vi "Tosca-Create And Enqueue Stimulus Rep.vi"(0 "Stim data in":T1, 1 "AODO Queue":refnum<queue>, 5 "Nreps":i32, 7 "Nqueue in":i32, 9 "Rep":i32, 11 "error in (no error)":errorcluster, 13 "tail":dbl[][](array[numeric])) -> (4 "Stim data out":T1, 8 "Nqueue out":i32, 15 "error out":errorcluster)   [LabVIEW 2020]
uses:
  Typedefs/Tosca-State AODO.ctl
  epl-vi-lib/Signal Synthesis VIs/4th Generation/Classes/SignalManager/SignalManager.lvclass
  Typedefs/Tosca-AO Runtime.ctl
  Typedefs/Tosca-DO Runtime.ctl
  Typedefs/Tosca-AODO Data.ctl
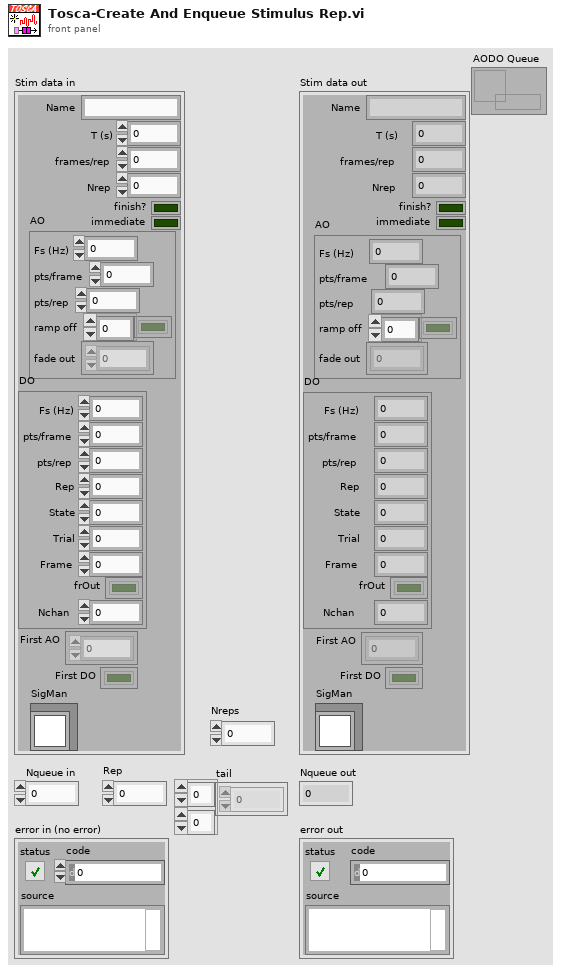
[diagram p1: front panel]
types:
  T1 = typedef "Tosca-State AODO.ctl" = cluster{"Name":string, "T (s)":dbl, "First AO":dbl[][], "frames/rep":i32, "finish?":bool, "Nrep":i32, "AO":T2, "DO":T3, "immediate":bool, "First DO":bool[][], "SigMan":refnum<class "SignalManager.lvclass">}
  T2 = typedef "Tosca-AO Runtime.ctl" = cluster{"Fs (Hz)":dbl, "pts/frame":i32, "pts/rep":i32, "ramp off":bool[], "fade out":dbl[][]}
  T3 = typedef "Tosca-DO Runtime.ctl" = cluster{"Fs (Hz)":dbl, "pts/frame":i32, "pts/rep":i32, "Rep":i32, "State":i32, "Trial":i32, "Frame":i32, "frOut":bool[], "Nchan":i32}
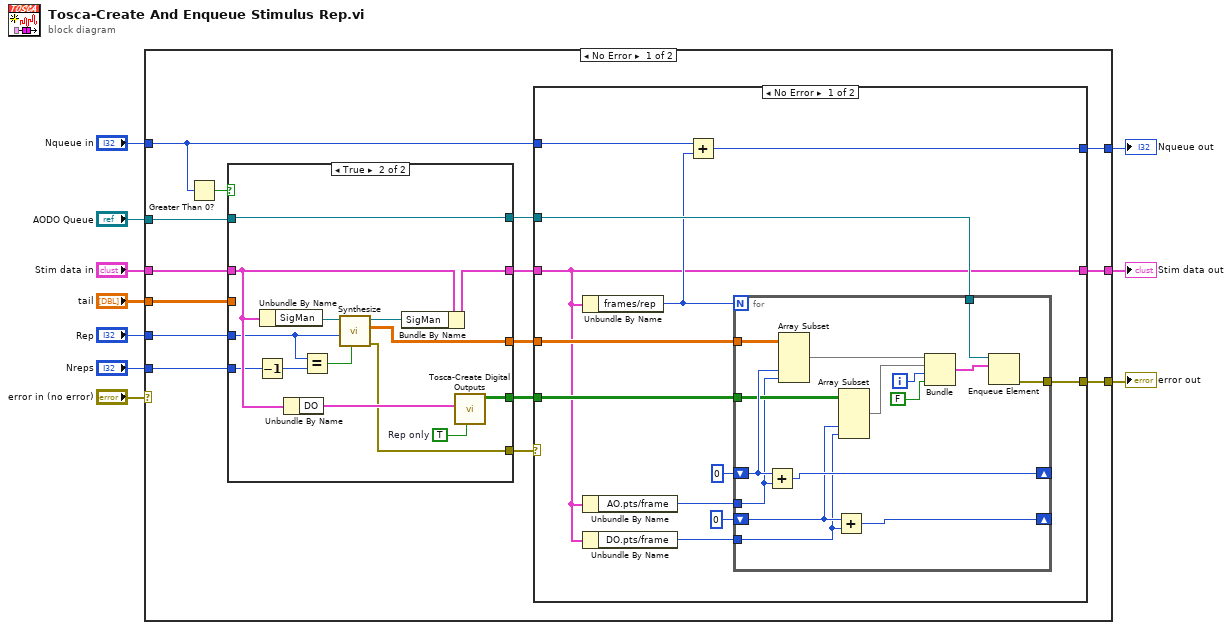
[diagram p0: block diagram]
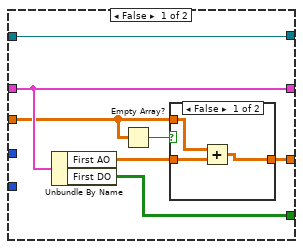
[diagram p3: hidden frame]
diagram:
  n1 = case shown="No Error" "error in (no error)" {
    selector: "error in (no error)" -> [_ w83]
    tunnel: "Stim data in" -> [w25 w81]
    tunnel: "Rep" -> [w24 _]
    tunnel: [w16 w81] -> w8
    tunnel: "AODO Queue" -> [w13 _]
    tunnel: "Nqueue in" -> [w20 w82]
    tunnel: [w19 w82] -> w5
    tunnel: [w18 w83] -> w4
    tunnel: "tail" -> [w12 _]
    tunnel: "Nreps" -> [w11 _]
    frame No Error {
      n2 = Greater Than 0?(x=w20) -> (x > 0?=w15:bool)
      n3 = case shown="True" w15 {
        tunnel: w25 -> [w60 w73]
        tunnel: [w56 w71] -> w23
        tunnel: [w62 w75] -> w21
        tunnel: [w60 w78] -> w22
        tunnel: [_ w74] -> w17
        tunnel: w24 -> [_ w70]
        tunnel: [w61 w72] -> w14
        tunnel: w13 -> [w61 w72]
        tunnel: w12 -> [w58 _]
        tunnel: w11 -> [_ w69]
        frame False {
          n4 = Unbundle By Name(w60) -> ("First AO"=w57:dbl[][], "First DO"=w62:bool[][])
          n5 = Empty Array?(array=w58) -> (empty?=w59:bool)
          n6 = case shown="False" w59 {
            tunnel: w58 -> [w64 _]
            tunnel: w57 -> [w65 w66]
            tunnel: [w63 w66] -> w56
            frame False {
              n7 = Add(x=w64, y=w65) -> (x+y=w63:dbl[][])
            }
            frame True {
            }
          }
        }
        frame True {
          w77 = TRUE  # Rep only
          n8 = Decrement(x=w69) -> (x-1=w68:i32)
          n9 = Unbundle By Name(w73) -> ("SigMan"=w80:refnum<class "SignalManager.lvclass">)
          n10 = Unbundle By Name(w73) -> ("DO"=w76:T3)
          n11 = Equal?(x=w70, y=w68) -> (x = y?=w67:bool)
          n12 = call "Synthesize.vi"("last"=w67, "Repetition"=w70, "SigMan in"=w80) -> ("error out"=w74:errorcluster, "Array"=w71:dbl[][], "SigMan out"=w79:refnum<class "SignalManager.lvclass">)  [unwired: 6 in]
          n13 = Bundle By Name(cluster=w73, "SigMan"=w79) -> (w78:T1)
          n14 = call "Tosca-Create Digital Outputs.vi"("Rep trigger only?"=w77, "DO"=w76) -> ("DO Array"=w75:bool[][])  [unwired: 8 in, 1 out]
        }
      }
      n15 = case shown="No Error" w17 {
        selector: w17 -> [_ w55]
        tunnel: w23 -> [w37 _]
        tunnel: w22 -> [w26 w53]
        tunnel: w21 -> [w32 _]
        tunnel: w14 -> [w31 _]
        tunnel: w20 -> [w30 w54]
        tunnel: [w28 w54] -> w19
        tunnel: [w27 w55] -> w18
        tunnel: [w26 w53] -> w16
        frame No Error {
          n16 = Unbundle By Name(w26) -> ("frames/rep"=w29:i32)
          n17 = Unbundle By Name(w26) -> ("AO.pts/frame"=w35:i32)
          n18 = Unbundle By Name(w26) -> ("DO.pts/frame"=w34:i32)
          n19 = Add(x=w30, y=w29) -> (x+y=w28:i32)
          n20 = for {
            N: w29 -> [_]
            tunnel: w37 -> [w52]
            shift-right: [w50] -> _
            shift-left: 0 -> [w51]
            tunnel: w35 -> [w46]
            tunnel: w34 -> [w45]
            shift-right: [w49] -> _
            shift-left: 0 -> [w47]
            tunnel: w32 -> [w48]
            tunnel: w31 -> [w41]
            tunnel: [w39] -> w27
            i -> [w42]
            n21 = Add(x=w51, y=w46) -> (x+y=w50:i32)
            n22 = Array Subset(array=w52, index (col)=w51, length (col)=w46) -> (w44:dbl[][])  [unwired: 2 in]
            n23 = Add(x=w47, y=w45) -> (x+y=w49:i32)
            n24 = Array Subset(array=w48, index (col)=w47, length (col)=w45) -> (w43:bool[][])  [unwired: 2 in]
            n25 = Bundle(w44, w43, w42, FALSE) -> (w40:cluster{dbl[][], bool[][], i32, bool})  [unwired: 1 in]
            n26 = Enqueue Element(queue=w41, element=w40) -> (error out=w39:errorcluster)  [unwired: 2 in, 2 out]
          }
        }
        frame Error {
        }
      }
    }
    frame Error {
    }
  }
  "Nqueue out" <- w5
  "error out" <- w4
  "Stim data out" <- w8
